vi "Get_Sweep_Speed.vi"(8 "error in (no error)":errorcluster, 11 ".NET Reference in":refnum<k24>) -> (0 "error out":errorcluster, 2 "speed out":dbl, 3 ".NET Reference out":refnum<k24>)   [LabVIEW 2017]
uses:
  LV_IL_Sample/DLL/InstrumentDLL.dll
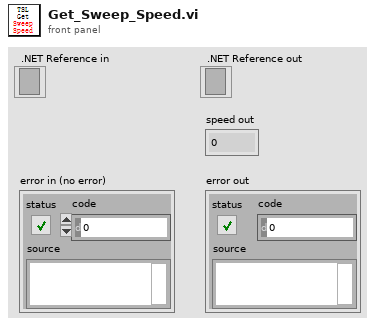
[diagram p1: front panel]
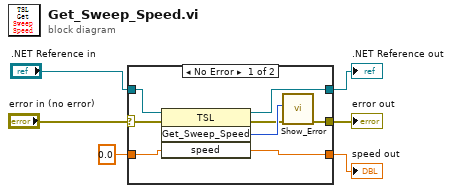
[diagram p0: block diagram]
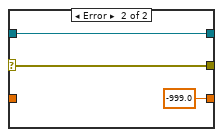
[diagram p2: hidden frame]
diagram:
  n1 = case shown="No Error" "error in (no error)" {
    selector: "error in (no error)" -> [w7 w17]
    tunnel: [w14 -999.0 ("speed")] -> w6
    tunnel: [w8 w17] -> w5
    tunnel: [w13 w15] -> w4
    tunnel: ".NET Reference in" -> [w12 w15]
    tunnel: 0.0 ("speed") -> [w11 _]
    frame No Error {
      n2 = invoke on="调用节点" class="TSL" method="Get_Sweep_Speed"(reference=w12, error in=w7, "speed"=w11) -> (reference out=w13:refnum<k24>, error out=w9:errorcluster, "Get_Sweep_Speed"=w10:i32, "speed"=w14:dbl)  [unwired: 1 in]
      n3 = call "Show_Error.vi"("error in (no error)"=w9, "Error"=w10) -> ("error out"=w8:errorcluster)  [unwired: 9 in]
    }
    frame Error {
    }
  }
  "speed out" <- w6
  "error out" <- w5
  ".NET Reference out" <- w4
